vi "Pickup Marker.vi"(8 "error in (no error)":errorcluster, 11 "Mouse in":refnum<class "Mouse.lvclass">) -> (0 "error out":errorcluster, 3 "Mouse out":refnum<class "Mouse.lvclass">)   [LabVIEW 2020, in "Maze.lvlib" / "Mouse.lvclass"]
doc: "Picks up a marker that has previously been placed with <b>Drop Marker.vi</b>. Using markers will score lower as it means an internal map is not being built within the mouse implementation."
uses:
  Mouse.lvclass
  Mouse.lvclass/Mouse.ctl
  Maze/Maze.lvclass
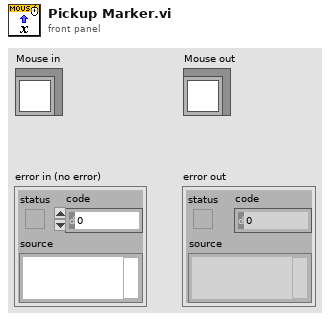
[diagram p1: front panel]
types:
  T1 = typedef "Maze.lvlib/Position.ctl" = cluster{"S":i32, "E":i32}
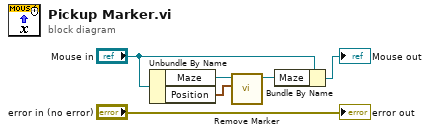
[diagram p0: block diagram]
diagram:
  n1 = Unbundle By Name("Mouse in") -> ("Maze"=w5:refnum<class "Maze.lvclass">, "Position"=w4:T1)
  n2 = call "Remove Marker.vi"("Position"=w4, "Maze in"=w5) -> ("Maze out"=w3:refnum<class "Maze.lvclass">)  [unwired: 8 in, 1 out]
  n3 = Bundle By Name(cluster="Mouse in", "Maze"=w3) -> (→"Mouse out":refnum<class "Mouse.lvclass">)
  "error out" <- "error in (no error)"
